vi "Test Reorder.vi"(8 "error in (no error)":errorcluster, 10 "Data Variant":variant, 11 "Reference Variant":variant) -> (0 "error out":errorcluster, 2 "Error":string, 3 "Output VData":variant)   [LabVIEW 2015]
uses:
  <vilib>/Utility/Data Type/NI_Data Type.lvlib
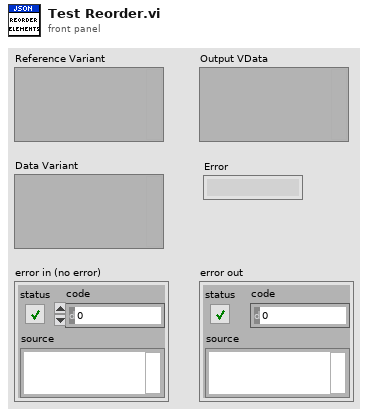
[diagram p1: front panel]
types:
  T1 = typedef "NI_Data Type.lvlib/Data Type.ctl" = enum8{"Invalid Type", "Void", "I8", "I16", "I32", "I64", "U8", "U16", "U32", "U64", "Single Float", "Double Float", "Extended Float", "Single Complex", "Double Complex", "Extended Complex", "Enum U8", "Enum U16", "Enum U32", "Enum U64", "Single Float With Unit", "Double Float With Unit", "Extended Float With Unit", "Single Complex with Unit", "Double Complex with Unit", "Extended Complex with Unit", "Boolean", "String", "Path", "Picture", "Tag", "Array", "Cluster", "Variant", "LV Variant", "Waveform", "Timestamp", "Digital Waveform", "Digital Data", "ExpressData", "Refnum", "External Data", "VI", "Poly VI", "LabVIEW Class Instance", "Fixed Point"}
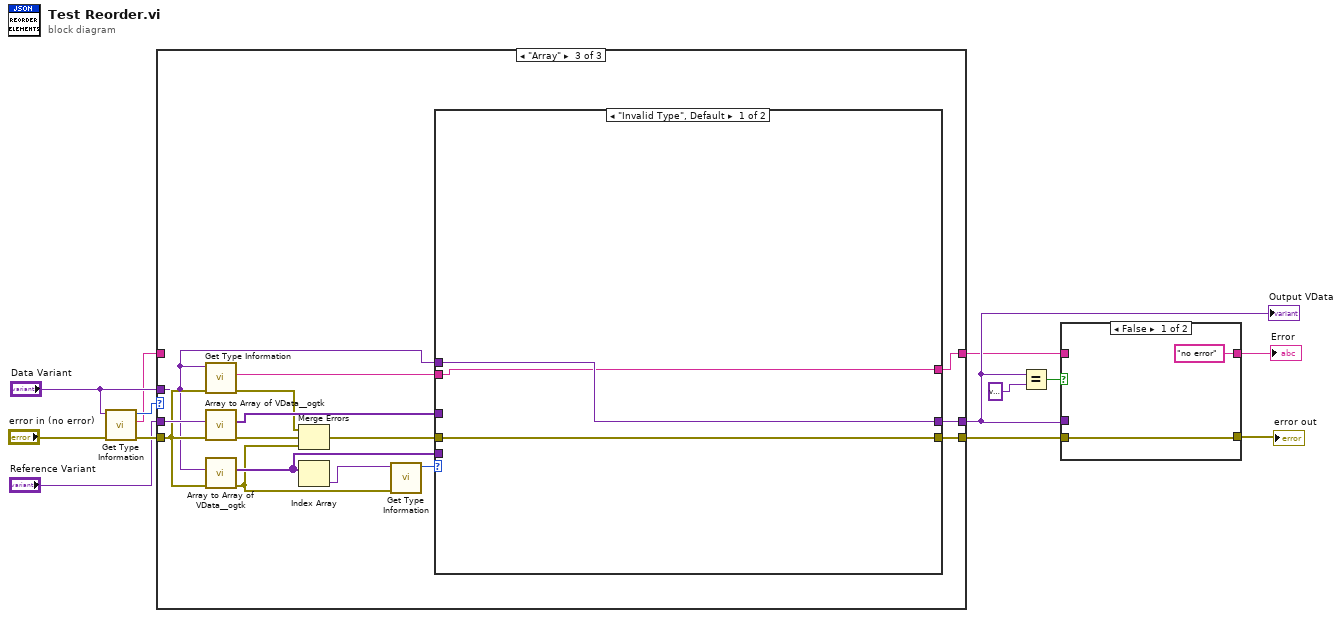
[diagram p0: block diagram]
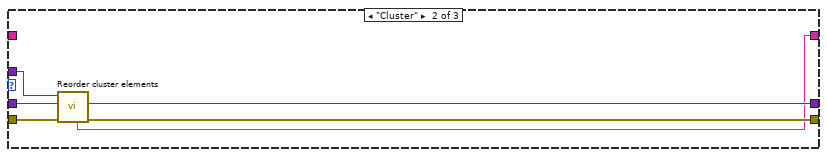
[diagram p4: hidden frame]
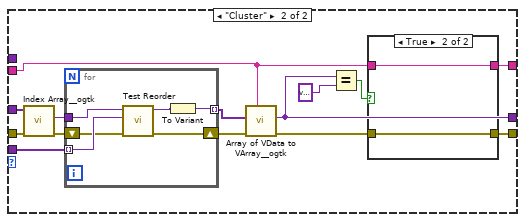
[diagram p5: hidden frame]
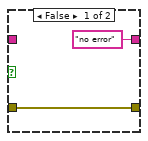
[diagram p6: hidden frame]
diagram:
  n1 = call <vilib>:"Get Type Information.vi"("error in (no error)"="error in (no error)", "Variant"="Data Variant") -> ("error out"=w13:errorcluster, "Name"=w3:string, "Type"=w12:T1)  [unwired: 5 in, 2 out]
  n2 = case shown="\"Array\"" w12 {
    tunnel: "Data Variant" -> [w16 w22 w25]
    tunnel: "Reference Variant" -> [_ w21 w37]
    tunnel: w13 -> [w15 w20 w32]
    tunnel: [w15 w19 w29] -> w5
    tunnel: [w16 w18 w30] -> w4
    tunnel: [w14 w17 w23] -> w2
    tunnel: w3 -> [w14 _ _]
    frame Default {
    }
    frame "Cluster" {
      n3 = call "Reorder cluster elements.vi"("error in (no error)"=w20, "Reference Variant"=w21, "Data Variant"=w22) -> ("error out"=w19:errorcluster, "Ordered VCluster"=w18:variant, "Current element name"=w17:string)  [unwired: 4 in, 2 out]
    }
    frame "Array" {
      n4 = call <vilib>:"Get Type Information.vi"("error in (no error)"=w32, "Variant"=w25) -> ("error out"=w31:errorcluster, "Name"=w33:string)  [unwired: 5 in, 3 out]
      n5 = call <userlib>:"Array to Array of VData__ogtk.vi"("error in (no error)"=w32, "MultiD Array"=w37) -> ("error out"=w35:errorcluster, "1D Array of Variants"=w36:variant[])  [unwired: 8 in]
      n6 = call <userlib>:"Array to Array of VData__ogtk.vi"("error in (no error)"=w32, "MultiD Array"=w25) -> ("error out"=w26:errorcluster, "1D Array of Variants"=w28:variant[])  [unwired: 8 in]
      n7 = Merge Errors(w31, w35, w26) -> (w34:errorcluster)
      n8 = Index Array(array=w28) -> (element=w27:variant)  [unwired: 1 in]
      n9 = call <vilib>:"Get Type Information.vi"("error in (no error)"=w26, "Variant"=w27) -> ("Type"=w24:T1)  [unwired: 5 in, 4 out]
      n10 = case shown="\"Invalid Type\", Default" w24 {
        tunnel: w36 -> [_ w54]
        tunnel: w34 -> [w39 w52]
        tunnel: w33 -> [w38 w42]
        tunnel: [w40 w45] -> w30
        tunnel: [w39 w43] -> w29
        tunnel: w28 -> [_ w49]
        tunnel: w25 -> [w40 _]
        tunnel: [w38 w41] -> w23
        frame "Invalid Type", Default {
        }
        frame "Cluster" {
          n11 = call <userlib>:"Index Array__ogtk.vi"("error in (no error)"=w52, "MultiD Array"=w54) -> ("error out"=w48:errorcluster, "Array Element"=w53:variant)  [unwired: 8 in]
          n12 = for {
            tunnel: w53 -> [w63]
            tunnel: w49 -> [w64] mode=indexing
            shift-right: [w61] -> w51
            shift-left: w48 -> [w62]
            tunnel: [w59] -> w50 mode=indexing
            n13 = call "Test Reorder.vi"("error in (no error)"=w62, "Data Variant"=w64, "Reference Variant"=w63) -> ("error out"=w61:errorcluster, "Output VData"=w60:variant)  [unwired: 6 in, 1 out]
            n14 = To Variant(anything=w60) -> (Variant=w59:variant)
          }
          n15 = call <userlib>:"Array of VData to VArray__ogtk.vi"("Array Name"=w42, "error in (no error)"=w51, "1D Array of VData"=w50) -> ("error out"=w44:errorcluster, "VArray"=w45:variant)  [unwired: 7 in]
          n16 = Equal?(x=w45, y=variant ("VArray")) -> (x = y?=w46:bool)
          n17 = case shown="True" w46 {
            tunnel: [w56 w57] -> w43
            tunnel: w44 -> [w56 w57]
            tunnel: w42 -> [_ w58]
            tunnel: ["no error" ("Name") w58] -> w41
            frame False {
            }
            frame True {
            }
          }
        }
      }
    }
  }
  "Output VData" <- w4
  n18 = Equal?(x=w4, y=variant ("VArray")) -> (x = y?=w9:bool)
  n19 = case shown="False" w9 {
    tunnel: w4 -> [_ _]
    tunnel: [w66 w67] -> w11
    tunnel: w5 -> [w66 w67]
    tunnel: w2 -> [_ w68]
    tunnel: ["no error" ("Name") w68] -> w1
    frame False {
    }
    frame True {
    }
  }
  "error out" <- w11
  "Error" <- w1
